vi "pipi.vi"() -> ()   [LabVIEW 2024]
panel:
  in  "stop":bool
  in  "Numérique":dbl
  in  "MDP":string
  in  "ID":string
  out "état":string
  in  "Déconnexion":bool
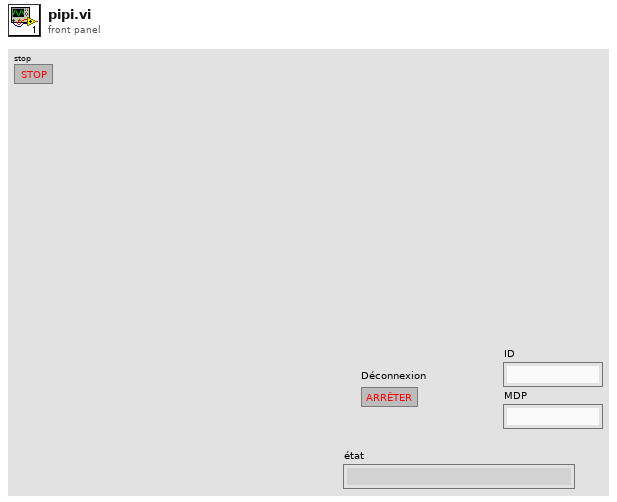
[diagram p1: front panel]
types:
  T1 = enum16{"Gerant", "Ressource Humaine", "Sécurité", "Finance", "Chef de Projet", "Chef de Ligne", "Salarié", "Déconnecter"}
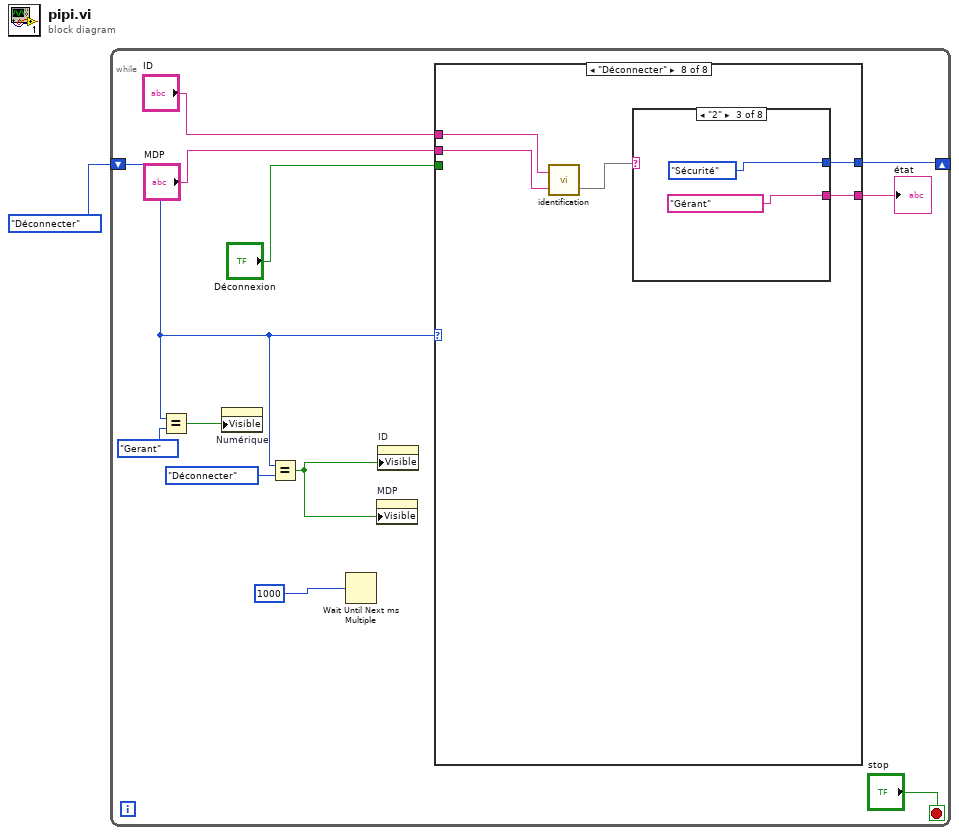
[diagram p0: block diagram]
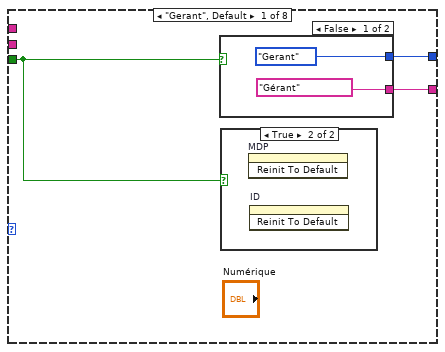
[diagram p2: hidden frame]
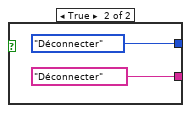
[diagram p4: hidden frame]
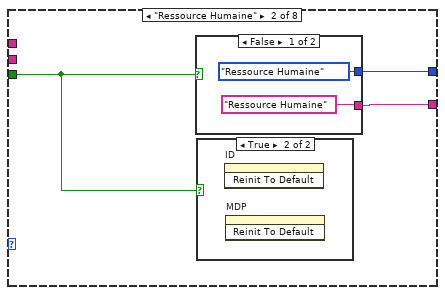
[diagram p5: hidden frame]
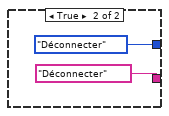
[diagram p7: hidden frame]
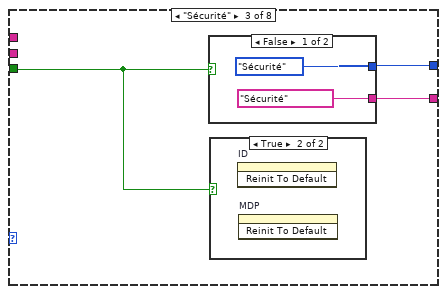
[diagram p8: hidden frame]
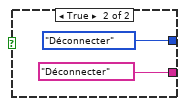
[diagram p10: hidden frame]
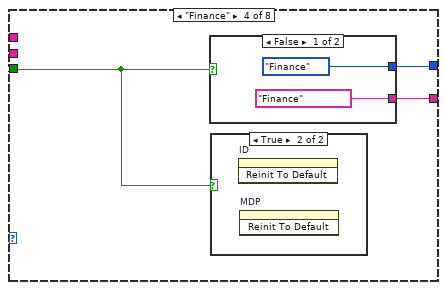
[diagram p11: hidden frame]
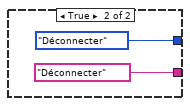
[diagram p13: hidden frame]
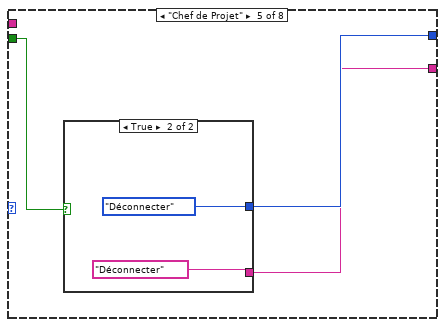
[diagram p14: hidden frame]
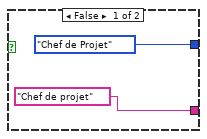
[diagram p15: hidden frame]
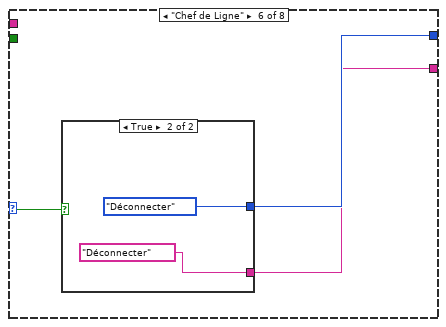
[diagram p16: hidden frame]
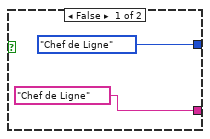
[diagram p17: hidden frame]
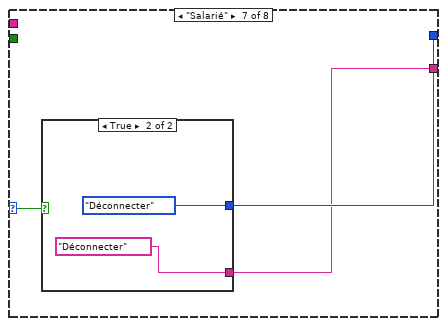
[diagram p18: hidden frame]
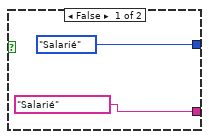
[diagram p19: hidden frame]
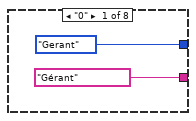
[diagram p20: hidden frame]
diagram:
  n1 = while {
    shift-right: [w13] -> _
    shift-left: T1."Déconnecter" -> [w4]
    stop <- "stop" stop-if-true
    n2 = Equal?(x=w4, y=T1."Gerant") -> (x = y?=w7:bool)
    n3 = property on="Numérique" class="DigNum (strict)"("Visible"=w7) -> ()  [unwired: 2 in, 2 out]
    n4 = Equal?(x=w4, y=T1."Déconnecter") -> (x = y?=w2:bool)
    n5 = Wait Until Next ms Multiple(millisecond multiple=1000) -> ()  [unwired: 1 out]
    n6 = property on="MDP" class="Str"("Visible"=w2) -> ()  [unwired: 2 in, 2 out]
    n7 = property on="ID" class="Str"("Visible"=w2) -> ()  [unwired: 2 in, 2 out]
    n8 = case shown="\"Déconnecter\"" w4 {
      tunnel: [w16 w23 w30 w37 w44 w50 w57 w67] -> w13
      tunnel: "Déconnexion" -> [w14 w21 w28 w35 w43 w51 w58 _]
      tunnel: [w15 w22 w29 w36 w42 w49 w56 w66] -> w11
      tunnel: "ID" -> [_ _ _ _ _ _ _ w65]
      tunnel: "MDP" -> [_ _ _ _ _ _ _ w64]
      frame "Gerant", Default {
        n9 = case shown="False" w14 {
          tunnel: [T1."Gerant" T1."Déconnecter"] -> w16
          tunnel: ["Gérant" "Déconnecter"] -> w15
          frame False {
          }
          frame True {
          }
        }
        n10 = case shown="True" w14 {
          frame False {
          }
          frame True {
            n11 = invoke on="MDP" class="Ch" method="Reinit To Default"() -> ()  [unwired: 3 in, 3 out]
            n12 = invoke on="ID" class="Ch" method="Reinit To Default"() -> ()  [unwired: 3 in, 3 out]
          }
        }
      }
      frame "Ressource Humaine" {
        n13 = case shown="False" w21 {
          tunnel: [T1."Ressource Humaine" T1."Déconnecter"] -> w23
          tunnel: ["Ressource Humaine" "Déconnecter"] -> w22
          frame False {
          }
          frame True {
          }
        }
        n14 = case shown="True" w21 {
          frame False {
          }
          frame True {
            n15 = invoke on="ID" class="Ch" method="Reinit To Default"() -> ()  [unwired: 3 in, 3 out]
            n16 = invoke on="MDP" class="Ch" method="Reinit To Default"() -> ()  [unwired: 3 in, 3 out]
          }
        }
      }
      frame "Sécurité" {
        n17 = case shown="False" w28 {
          tunnel: [T1."Sécurité" T1."Déconnecter"] -> w30
          tunnel: ["Sécurité" "Déconnecter"] -> w29
          frame False {
          }
          frame True {
          }
        }
        n18 = case shown="True" w28 {
          frame False {
          }
          frame True {
            n19 = invoke on="ID" class="Ch" method="Reinit To Default"() -> ()  [unwired: 3 in, 3 out]
            n20 = invoke on="MDP" class="Ch" method="Reinit To Default"() -> ()  [unwired: 3 in, 3 out]
          }
        }
      }
      frame "Finance" {
        n21 = case shown="False" w35 {
          tunnel: [T1."Finance" T1."Déconnecter"] -> w37
          tunnel: ["Finance" "Déconnecter"] -> w36
          frame False {
          }
          frame True {
          }
        }
        n22 = case shown="True" w35 {
          frame False {
          }
          frame True {
            n23 = invoke on="ID" class="Ch" method="Reinit To Default"() -> ()  [unwired: 3 in, 3 out]
            n24 = invoke on="MDP" class="Ch" method="Reinit To Default"() -> ()  [unwired: 3 in, 3 out]
          }
        }
      }
      frame "Chef de Projet" {
        n25 = case shown="True" w43 {
          tunnel: [T1."Chef de Projet" T1."Déconnecter"] -> w44
          tunnel: ["Chef de projet" "Déconnecter"] -> w42
          frame False {
          }
          frame True {
          }
        }
      }
      frame "Chef de Ligne" {
        n26 = case shown="True" w51 {
          tunnel: [T1."Chef de Ligne" T1."Déconnecter"] -> w50
          tunnel: ["Chef de Ligne" "Déconnecter"] -> w49
          frame False {
          }
          frame True {
          }
        }
      }
      frame "Salarié" {
        n27 = case shown="True" w58 {
          tunnel: [T1."Salarié" T1."Déconnecter"] -> w57
          tunnel: ["Salarié" "Déconnecter"] -> w56
          frame False {
          }
          frame True {
          }
        }
      }
      frame "Déconnecter" {
        n28 = call "identification.vi"("Password"=w64, "Identifiant"=w65) -> (0:w63)  [unwired: 1 out]
        n29 = case shown="\"2\"" w63 {
          tunnel: [T1."Gerant" T1."Ressource Humaine" T1."Sécurité" T1."Finance" T1."Chef de Projet" T1."Chef de Ligne" T1."Salarié" T1."Déconnecter"] -> w67
          tunnel: ["Gérant" "Ressource Humaine" "Gérant" "Gérant" "Gérant" "Gérant" "Gérant" "Déconnecter"] -> w66
          frame "0" {
          }
          frame "1" {
          }
          frame "2" {
          }
          frame "3" {
          }
          frame "4" {
          }
          frame "5" {
          }
          frame "6" {
          }
          frame "7", Default {
          }
        }
      }
    }
    "état" <- w11
  }
